vi "Async-Or-Show.GetAutotoolRegionsRuntime.vi"(0 "XRef":T9, 1 "State In":T6) -> (14 "Regions":T1)   [LabVIEW 2015, in "Async-Or-Show.xnode"]
uses:
  Async-Or-Show.xnode
  <vilib>/XNodeSupport/XNodeXNodeRef.ctl
  State.ctl
  <vilib>/Utility/miscctls.llb/LVRectTypeDef.ctl
  <vilib>/picture/picture.llb/imagedata.ctl
  <vilib>/XNodeSupport/XNodeAutotoolRegions.ctl
  <vilib>/XNodeSupport/XNodeAutotoolRegion.ctl
  <vilib>/XNodeSupport/XNodeRect32.ctl
  <vilib>/XNodeSupport/XNodeInt.ctl
  <vilib>/XNodeSupport/XNodeTools.ctl
  <vilib>/XNodeSupport/NI_XNodeSupport.lvlib
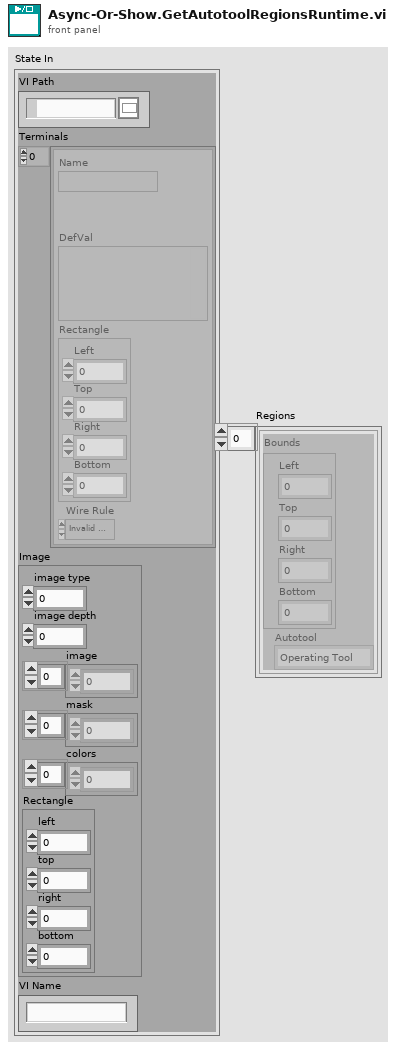
[diagram p1: front panel]
types:
  T1 = typedef "NI_XNodeSupport.lvlib/XNodeAutotoolRegions.ctl" = T2[]
  T2 = typedef "NI_XNodeSupport.lvlib/XNodeAutotoolRegion.ctl" = cluster{"Bounds":T3, "Autotool":T5}
  T3 = typedef "NI_XNodeSupport.lvlib/XNodeRect32.ctl" = cluster{"Left":T4, "Top":T4, "Right":T4, "Bottom":T4}
  T4 = typedef "NI_XNodeSupport.lvlib/XNodeInt.ctl" = i32
  T5 = typedef "NI_XNodeSupport.lvlib/XNodeTools.ctl" = enum32{"Operating Tool", "Placement Tool", "Labelling Tool", "Wiring Tool", "Scroll Tool", "Breakpoint Tool", "Probe Tool", "Auto Tool"}
  T6 = typedef "Async-Or-Show.xnode/State.ctl" = cluster{"VI Path":path, "Terminals":cluster{"Name":string, "DefVal":variant, "Rectangle":T7, "Wire Rule":enum16{"Invalid Wire Rule", "Required", "Recommended", "Optional", "Dynamic Dispatch"}}[], "Image":T8, "VI Name":string}
  T7 = typedef "LVRectTypeDef.ctl" = cluster{"Left":i16, "Top":i16, "Right":i16, "Bottom":i16}
  T8 = typedef "imagedata.ctl" = cluster{"image type":i32, "image depth":i32, "image":u8[], "mask":u8[], "colors":u32[], "Rectangle":cluster{"left":i16, "top":i16, "right":i16, "bottom":i16}}
  T9 = typedef "NI_XNodeSupport.lvlib/XNodeXNodeRef.ctl" = refnum<vi>
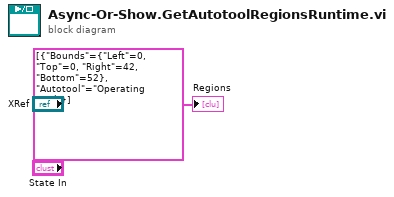
[diagram p0: block diagram]
diagram:
  "Regions" <- T1 [{"Bounds"={"Left"=0, "Top"=0, "Right"=42, "Bottom"=52}, "Autotool"=enum."Operating Tool"}] ("Regions")
